vi "lib XML Section.vi"(8 "error in (no error)":errorcluster, 10 "XML String":string, 11 "XML Topic":string) -> (0 "error out":errorcluster, 1 "after substring":string, 2 "XML Topic Body":string, 3 "XML Topic dup":string)   [LabVIEW 2024]
uses:
  <vilib>/Utility/error.llb/Trim Whitespace One-Sided.vi
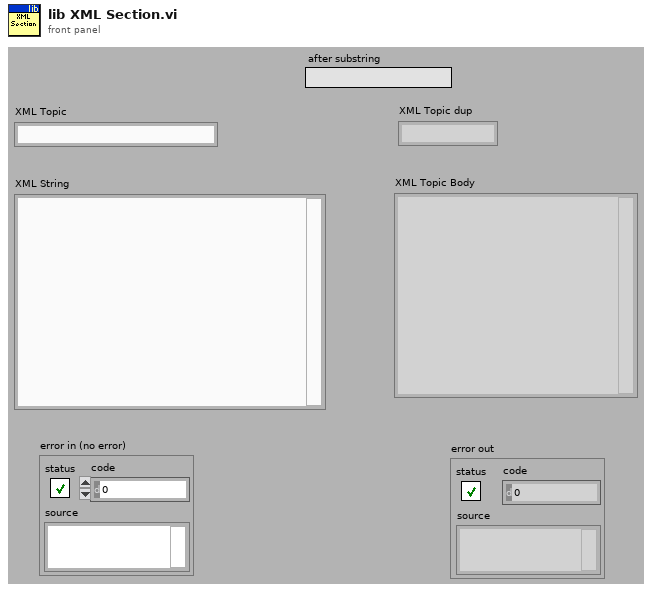
[diagram p1: front panel]
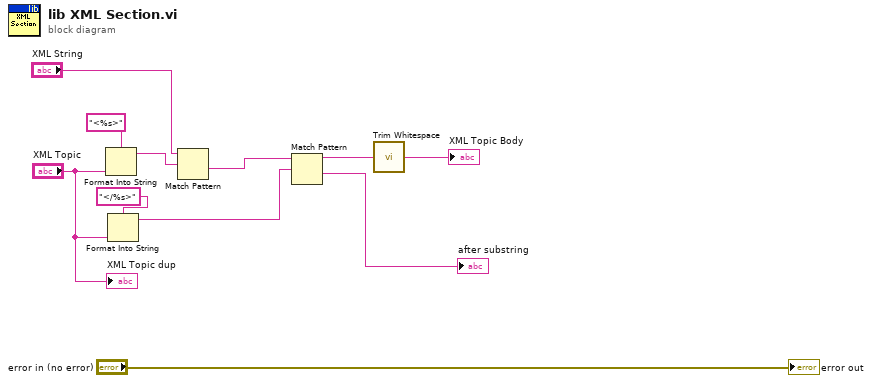
[diagram p0: block diagram]
diagram:
  n1 = Format Into String(format string="<%s>", "XML Topic") -> (resulting string=w8:string)  [unwired: 2 in, 1 out]
  n2 = Format Into String(format string="</%s>", "XML Topic") -> (resulting string=w6:string)  [unwired: 2 in, 1 out]
  n3 = Match Pattern(string="XML String", regular expression=w8) -> (after substring=w5:string)  [unwired: 1 in, 3 out]
  n4 = Match Pattern(string=w5, regular expression=w6) -> (before substring=w4:string, after substring=→"after substring":string)  [unwired: 1 in, 2 out]
  n5 = call <vilib>:"Trim Whitespace.vi"("string"=w4) -> ("trimmed string"=→"XML Topic Body":string)  [unwired: 1 in]
  "error out" <- "error in (no error)"
  "XML Topic dup" <- "XML Topic"
